vi "SerialPortTest.vi"() -> ()   [LabVIEW 2013]
panel:
  out "Num Bytes Written":u32
  out "error out 2":errorcluster
  out "error out":errorcluster
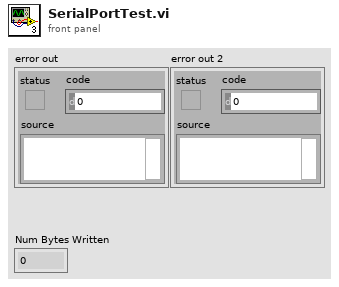
[diagram p1: front panel]
types:
  T1 = typedef "WPI_SerialPortRef.ctl" = cluster{"DevStatus":errorcluster, "Serial Port Name":refnum<visa-resource-name>}
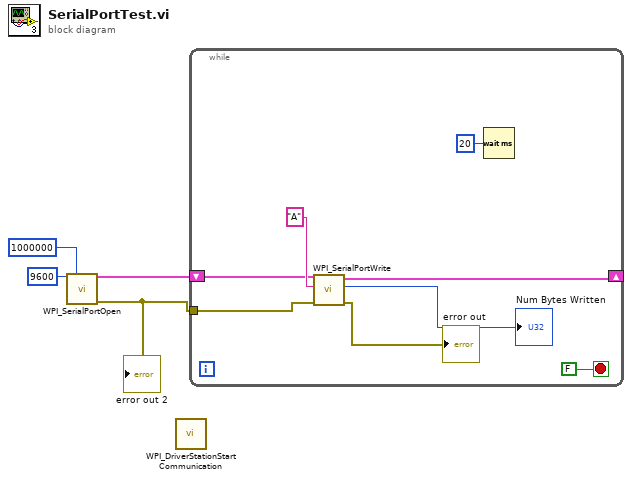
[diagram p0: block diagram]
diagram:
  n1 = call <vilib>:"WPI_SerialPortOpen.vi"("Baud Rate"=u32 9600, "Timeout Value (ms)"=u32 1000000) -> ("SerialPortRef"=w4:T1, "error out"=w3:errorcluster)  [unwired: 12 in]
  "error out 2" <- w3
  n2 = call <vilib>:"WPI_DriverStationStart Communication.vi"() -> ()  [unwired: 12 in]
  n3 = while {
    tunnel: w3 -> [w6]
    shift-right: [w8] -> _
    shift-left: w4 -> [w9]
    stop <- FALSE stop-if-true
    n4 = call <vilib>:"WPI_SerialPortWrite.vi"("error in (no error)"=w6, "Buffer"="A", "SerialPortRef"=w9) -> ("error out"=→"error out":errorcluster, "Num Bytes Written"=→"Num Bytes Written":u32, "SerialPortRef"=w8:T1)  [unwired: 6 in]
    n5 = Wait (ms)(milliseconds to wait=u32 20) -> ()  [unwired: 1 out]
  }
